vi "Configure Measurement Function.vi"(8 "error in (no error)":errorcluster, 10 "Function (0: Volts)":u16(ring) items=["Volts", "Current", "Auto Resistance", "Manual Resistance", "Digitize Voltage", "Digitize Current"], 11 "VISA resource name":refnum<visa-resource-name>) -> (0 "error out":errorcluster, 3 "VISA resource name out":refnum<visa-resource-name>)   [LabVIEW 2016, in "Keithley 2450.lvlib"]
doc: "Configures the measurement function on the instrument."
uses:
  Keithley 2450.lvlib
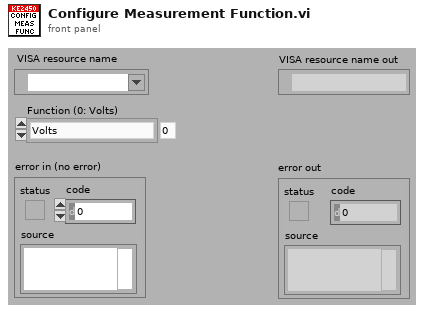
[diagram p1: front panel]
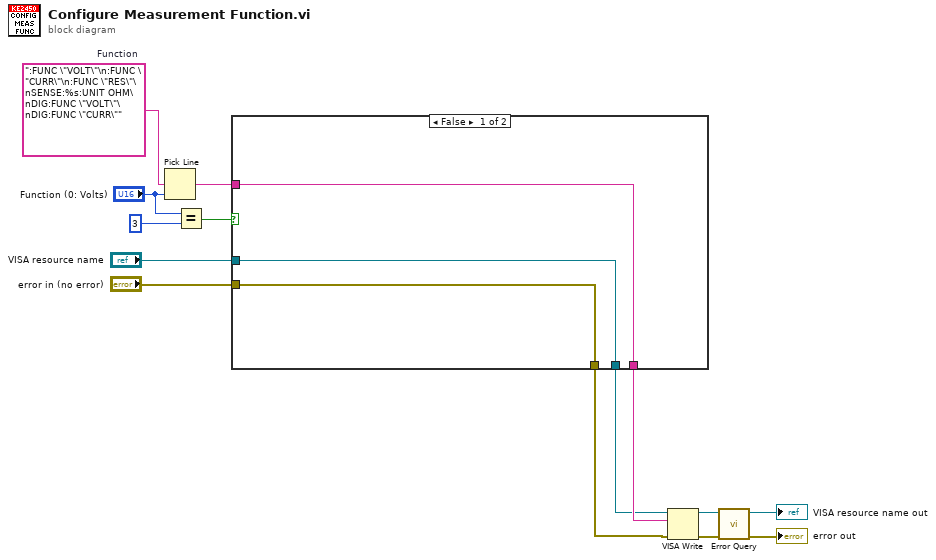
[diagram p0: block diagram]
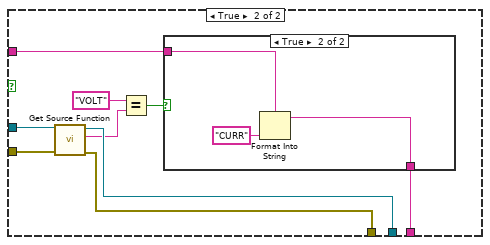
[diagram p2: hidden frame]
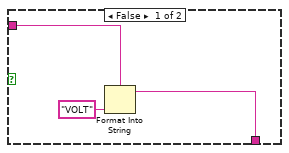
[diagram p3: hidden frame]
diagram:
  w12 = ":FUNC \"VOLT\"\n:FUNC \"CURR\"\n:FUNC \"RES\"\nSENSE:%s:UNIT OHM\nDIG:FUNC \"VOLT\"\nDIG:FUNC \"CURR\""  # Function
  n1 = Pick Line(multi-line string=w12, line index="Function (0: Volts)") -> (output string=w5:string)  [unwired: 1 out]
  n2 = Equal?(x="Function (0: Volts)", y=u16 3) -> (x = y?=w7:bool)
  n3 = case shown="False" w7 {
    tunnel: [w17 w18] -> w6
    tunnel: w5 -> [w17 w19]
    tunnel: "VISA resource name" -> [w16 w26]
    tunnel: "error in (no error)" -> [w15 w25]
    tunnel: [w16 w24] -> w2
    tunnel: [w15 w23] -> w1
    frame False {
    }
    frame True {
      n4 = call "Get Source Function.vi"("error in (no error)"=w25, "VISA resource name"=w26) -> ("error out"=w23:errorcluster, "Source Function"=w22:string, "VISA resource name out"=w24:refnum<visa-resource-name>)  [unwired: 7 in]
      n5 = Equal?(x="VOLT", y=w22) -> (x = y?=w20:bool)
      n6 = case shown="True" w20 {
        tunnel: w19 -> [w28 w31]
        tunnel: [w27 w30] -> w18
        frame False {
          n7 = Format Into String(format string=w28, "VOLT" ("input 1")) -> (resulting string=w27:string)  [unwired: 2 in, 1 out]
        }
        frame True {
          n8 = Format Into String(format string=w31, "CURR" ("input 1")) -> (resulting string=w30:string)  [unwired: 2 in, 1 out]
        }
      }
    }
  }
  n9 = VISA Write(VISA resource name=w2, write buffer=w6, error in (no error)=w1) -> (VISA resource name out=w11:refnum<visa-resource-name>, error out=w10:errorcluster)  [unwired: 1 out]
  n10 = call "Error Query.vi"("error in (no error)"=w10, "VISA resource name"=w11) -> ("error out"=→"error out":errorcluster, "VISA resource name out"=→"VISA resource name out":refnum<visa-resource-name>)  [unwired: 8 out]
